vi "NicmosSerial.vi"(0 "error in":errorcluster, 2 "timeout (10sec)":i32=-1 caption="Timeout (-1)", 5 "Command":string) -> (3 "error out":errorcluster, 6 "Answer":string)   [LabVIEW 2009]
uses:
  NicmosGlobal.vi
  <vilib>/Instr/_visa.llb/VISA Configure Serial Port (Serial Instr).vi
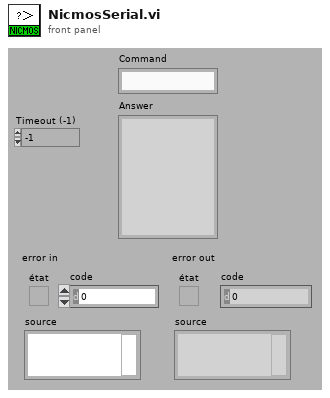
[diagram p1: front panel]
types:
  T1 = typedef "Semaphore RefNum" = refnum<k1>
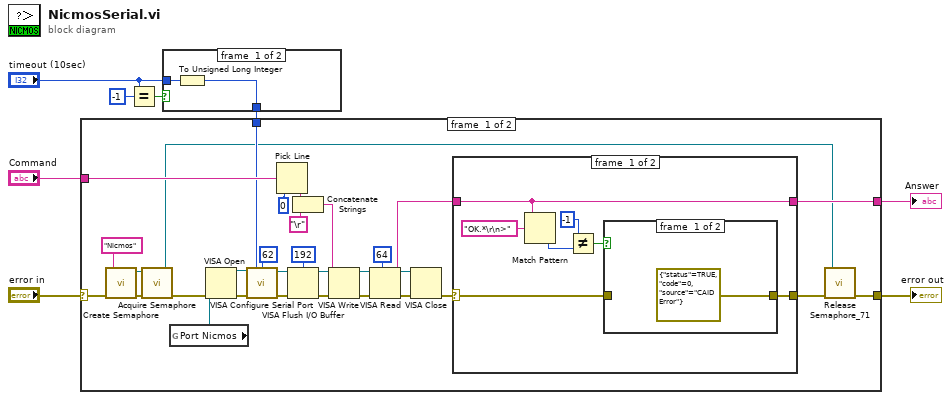
[diagram p0: block diagram]
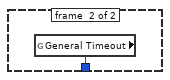
[diagram p2: hidden frame]
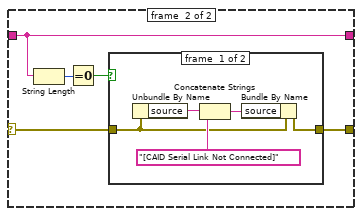
[diagram p4: hidden frame]
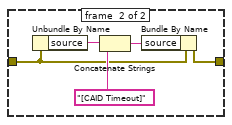
[diagram p5: hidden frame]
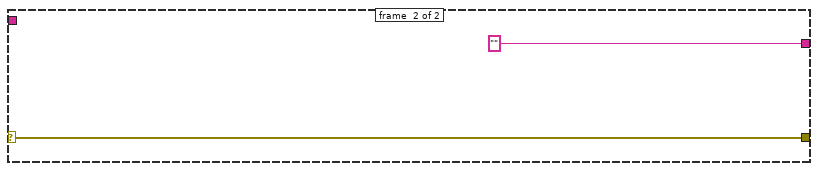
[diagram p6: hidden frame]
diagram:
  n1 = Equal?(x="timeout (10sec)", y=-1) -> (x = y?=w4:bool)
  n2 = case shown="True" w4 {
    tunnel: [w9 w11] -> w3
    tunnel: "timeout (10sec)" -> [w10 _]
    frame #0 {
      n3 = To Unsigned Long Integer(number=w10) -> (unsigned 32bit integer=w9:u32)
    }
    frame #1 {
      n4 = global read "NicmosGlobal.vi" "General Timeout"() -> (w11:u32)
    }
  }
  n5 = case shown="No Error" "error in" {
    selector: "error in" -> [w35 w68]
    tunnel: "Command" -> [w39 _]
    tunnel: [w30 w68] -> w1
    tunnel: [w38 "" ("read buffer")] -> w8
    tunnel: w3 -> [w36 _]
    frame #0 {
      n6 = call <vilib>:"Create Semaphore.vi"("error in (no error)"=w35, "name (unnamed)"="Nicmos") -> ("error out"=w34:errorcluster, "semaphore"=w32:T1)  [unwired: 3 in, 1 out]
      n7 = call <vilib>:"Acquire Semaphore.vi"("error in (no error)"=w34, "semaphore"=w32) -> ("error out"=w20:errorcluster, "semaphore out"=w29:T1)  [unwired: 3 in, 1 out]
      n8 = global read "NicmosGlobal.vi" "Port Nicmos"() -> (w12:refnum<visa-resource-name>)
      n9 = VISA Open(error in (no error)=w20, VISA resource name=w12) -> (VISA resource name=w18:refnum<visa-resource-name>, error out=w19:errorcluster)  [unwired: 3 in]
      n10 = call-poly "VISA Configure Serial Port"("VISA resource name"=w18, "timeout (10sec)"=w36, "termination char\n(0xA = '\\n' = LF)"=u8 62 ("termination char\n(0xA = '\\n' = LF)"), "error in (no error)"=w19) -> ("VISA resource name out"=w26:refnum<visa-resource-name>, "error out"=w25:errorcluster)  [unwired: 10 in]
      n11 = Pick Line(multi-line string=w39, line index=0 ("indice de ligne")) -> (output string=w40:string)  [unwired: 1 in]
      n12 = VISA Flush I/O Buffer(VISA resource name=w26, mask (16)=u16 192 ("masque (16)"), error in (no error)=w25) -> (VISA resource name out=w24:refnum<visa-resource-name>, error out=w23:errorcluster)
      n13 = Concatenate Strings(w40, "\r") -> (w37:string)
      n14 = VISA Write(VISA resource name=w24, write buffer=w37, error in (no error)=w23) -> (VISA resource name out=w17:refnum<visa-resource-name>, error out=w22:errorcluster)  [unwired: 1 out]
      n15 = VISA Read(VISA resource name=w17, byte count=u32 64 ("nombre d'octets (0)"), error in (no error)=w22) -> (VISA resource name out=w15:refnum<visa-resource-name>, read buffer=w13:string, error out=w16:errorcluster)  [unwired: 1 out]
      n16 = VISA Close(VISA resource name=w15, error in (no error)=w16) -> (error out=w14:errorcluster)
      n17 = case shown="No Error" w14 {
        selector: w14 -> [w44 w52]
        tunnel: w13 -> [w43 w54]
        tunnel: [w45 w53] -> w31
        tunnel: [w43 w54] -> w38
        frame #0 {
          n18 = Match Pattern(string=w43, regular expression="OK.*\r\n>" ("expression")) -> (offset past match=w48:i32)  [unwired: 1 in, 3 out]
          n19 = Not Equal?(x=-1, y=w48) -> (x != y?=w46:bool)
          n20 = case shown="True" w46 {
            tunnel: w44 -> [_ w51]
            tunnel: [errorcluster {"status"=TRUE, "code"=0, "source"="CAID Error"} ("error out") w51] -> w45
            frame #0 {
            }
            frame #1 {
            }
          }
        }
        frame #1 {
          n21 = String Length(string=w54) -> (length=w56:i32)
          n22 = Equal To 0?(x=w56) -> (x = 0?=w55:bool)
          n23 = case shown="True" w55 {
            tunnel: [w57 w62] -> w53
            tunnel: w52 -> [w58 w63]
            frame #0 {
              n24 = Unbundle By Name(w58) -> ("source"=w61:string)
              n25 = Concatenate Strings(w61, "[CAID Serial Link Not Connected]" ("source")) -> (w59:string)
              n26 = Bundle By Name(cluster=w58, "source"=w59) -> (w57:errorcluster)
            }
            frame #1 {
              n27 = Unbundle By Name(w63) -> ("source"=w66:string)
              n28 = Concatenate Strings(w66, "[CAID Timeout]" ("source")) -> (w64:string)
              n29 = Bundle By Name(cluster=w63, "source"=w64) -> (w62:errorcluster)
            }
          }
        }
      }
      n30 = call <vilib>:"Release Semaphore_71.vi"("error in (no error)"=w31, "semaphore"=w29) -> ("error out"=w30:errorcluster)  [unwired: 4 in, 1 out]
    }
    frame #1 {
    }
  }
  "error out" <- w1
  "Answer" <- w8
